vi "Routine.vi"(11 "TEMPLATE jettl in":refnum<class "TEMPLATE jettl.lvclass">) -> (3 "TEMPLATE jettl out":refnum<class "TEMPLATE jettl.lvclass">)   [LabVIEW 2021, in "_Template.lvlib" / "Templates.lvlib" / "TEMPLATE jettl.lvlib" / "TEMPLATE jettl.lvclass"]
uses:
  TEMPLATE jettl.lvclass
  C:/git/jettl/jettl/jettl/jettl/jettl.lvclass
  TEMPLATE jettl.lvclass/TEMPLATE jettl.ctl
  jettl/jettl/jettl/jettl.lvclass
  jettl/jettl/Msg Strategy/Msg Strategy.lvclass
panel:
  # "Note the VI Properties have been modified for typical UI window settings.\n\nThis panel operates as a normal user interface.\nClick the Panel Close? for the default implemention to occur: executing the Teardown method."
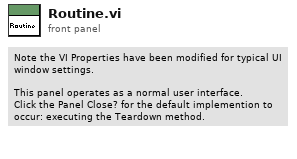
[diagram p1: front panel]
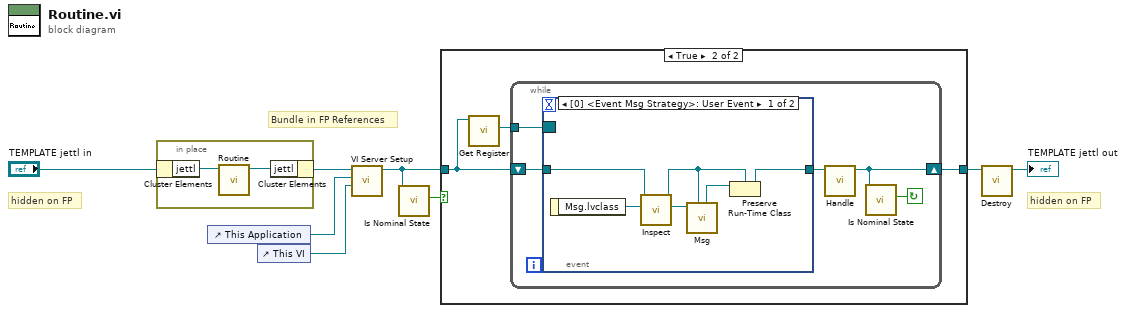
[diagram p0: block diagram]
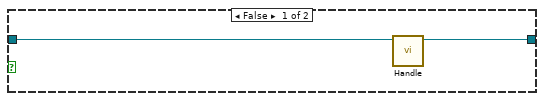
[diagram p2: hidden frame]
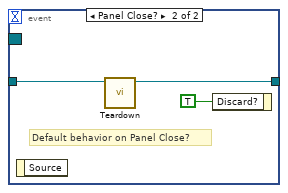
[diagram p3: hidden frame]
diagram:
  # "Bundle in FP References"
  # "hidden on FP"
  # "hidden on FP"
  n1 = in-place {
    n2 = in-place-cluster #1("TEMPLATE jettl in") -> ("jettl"=w10:refnum<class "jettl.lvclass">)
    n3 = call-dynamic "Routine.vi"("jettl in"=w10) -> ("jettl out"=w9:refnum<class "jettl.lvclass">)  [unwired: 10 in]
    n4 = in-place-cluster #1("jettl"=w9) -> (w3:refnum<class "TEMPLATE jettl.lvclass">)
  }
  n5 = control-ref of="This Application"() -> (w2:refnum<vi>)
  n6 = control-ref of="This VI"() -> (w1:refnum<vi>)
  n7 = call-dynamic "VI Server Setup.vi"("This VI"=w1, "This Application"=w2, "TEMPLATE jettl in"=w3) -> ("TEMPLATE jettl out"=w5:refnum<class "TEMPLATE jettl.lvclass">)  [unwired: 8 in]
  n8 = call-dynamic "Is Nominal State.vi"("TEMPLATE jettl in"=w5) -> ("Is Nominal State?"=w4:bool)  [unwired: 10 in]
  n9 = case shown="True" w4 {
    tunnel: w5 -> [w12 w13]
    tunnel: [w11 w15] -> w7
    frame False {
      n10 = call-dynamic "Handle.vi"("TEMPLATE jettl in"=w12) -> ("TEMPLATE jettl out"=w11:refnum<class "TEMPLATE jettl.lvclass">)  [unwired: 10 in]
    }
    frame True {
      n11 = call-dynamic "Get Register.vi"("TEMPLATE jettl in"=w13) -> ("Register"=w14:refnum<event-registration>)  [unwired: 10 in]
      n12 = while {
        shift-right: [w17] -> w15
        shift-left: w13 -> [w19]
        tunnel: w14 -> [w20]
        stop <- w16 continue-if-true
        n13 = event shown="[0] <Event Msg Strategy>: User Event" {
          selector: w20 -> [_ _]
          dyn-events: _ -> [_ _]
          timeout: _ -> [_ _]
          tunnel: w19 -> [w21 w28]
          tunnel: [w26 w27] -> w18
          event User Event {
            n14 = event-data() -> ("Msg.lvclass"=w24:refnum<class "Msg Strategy.lvclass">)  [unwired: 1 in]
            n15 = call-dynamic "Inspect.vi"("Msg Strategy in"=w24, "TEMPLATE jettl in"=w21) -> ("Msg Strategy out"=w23:refnum<class "Msg Strategy.lvclass">, "TEMPLATE jettl out"=w22:refnum<class "TEMPLATE jettl.lvclass">)  [unwired: 8 in]
            n16 = call-dynamic "Msg.vi"("jettl in"=w22, "Msg Strategy in"=w23) -> ("jettl out"=w25:refnum<class "jettl.lvclass">)  [unwired: 9 in]
            n17 = Preserve Run-Time Class(object in=w25, 2:w22) -> (object out=w26:refnum<class "TEMPLATE jettl.lvclass">)  [unwired: 1 in, 1 out]
          }
          event Panel Close? {
            # "Default behavior on Panel Close?"
            n18 = event-data() -> ()  [unwired: 1 in, 1 out]
            n19 = call-dynamic "Teardown.vi"("TEMPLATE jettl in"=w28) -> ("TEMPLATE jettl out"=w27:refnum<class "TEMPLATE jettl.lvclass">)  [unwired: 10 in]
            n20 = event-data("Discard?"=TRUE) -> ()  [unwired: 1 in, 1 out]
          }
        }
        n21 = call-dynamic "Handle.vi"("TEMPLATE jettl in"=w18) -> ("TEMPLATE jettl out"=w17:refnum<class "TEMPLATE jettl.lvclass">)  [unwired: 10 in]
        n22 = call-dynamic "Is Nominal State.vi"("TEMPLATE jettl in"=w17) -> ("Is Nominal State?"=w16:bool)  [unwired: 10 in]
      }
    }
  }
  n23 = call-dynamic "Destroy.vi"("TEMPLATE jettl in"=w7) -> ("TEMPLATE jettl out"=→"TEMPLATE jettl out":refnum<class "TEMPLATE jettl.lvclass">)  [unwired: 10 in]
